vi "test BNR and BCD Parameters that Span Words.vi"(8 "error in":errorcluster, 11 "Loopback in":refnum<class "Loopback.lvclass">) -> (0 "error out":errorcluster, 3 "Loopback out":refnum<class "Loopback.lvclass">)   [LabVIEW 2020, in "Loopback.lvclass"]
uses:
  Loopback.lvclass
  C:/Users/nitest/Desktop/Git 2020/niveristand-custom-device-testing-tools/VeriStandTestCase/VeriStandTestCase.lvclass
  niveristand-custom-device-testing-tools/VeriStandTestUtilities/VeriStandTestUtilities.lvlib
  <vilib>/addons/_JKI Toolkits/VI Tester/TestCase.llb/TestCase.lvclass
  C:/Program Files (x86)/National Instruments/LabVIEW 2020/vi.lib/addons/_JKI Toolkits/VI Tester/TestCase.llb/TestCase.lvclass
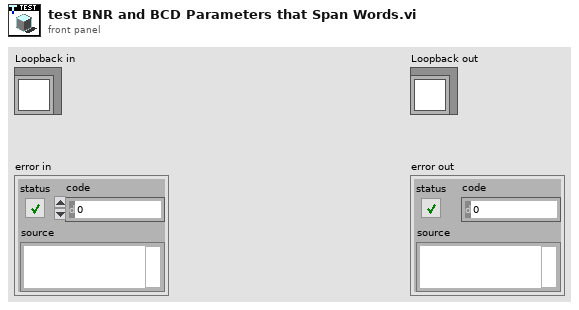
[diagram p1: front panel]
types:
  T1 = typedef "NI_VS Workspace ExecutionAPI.lvlib/WorkspaceAPI.ctl" = refnum<k24>
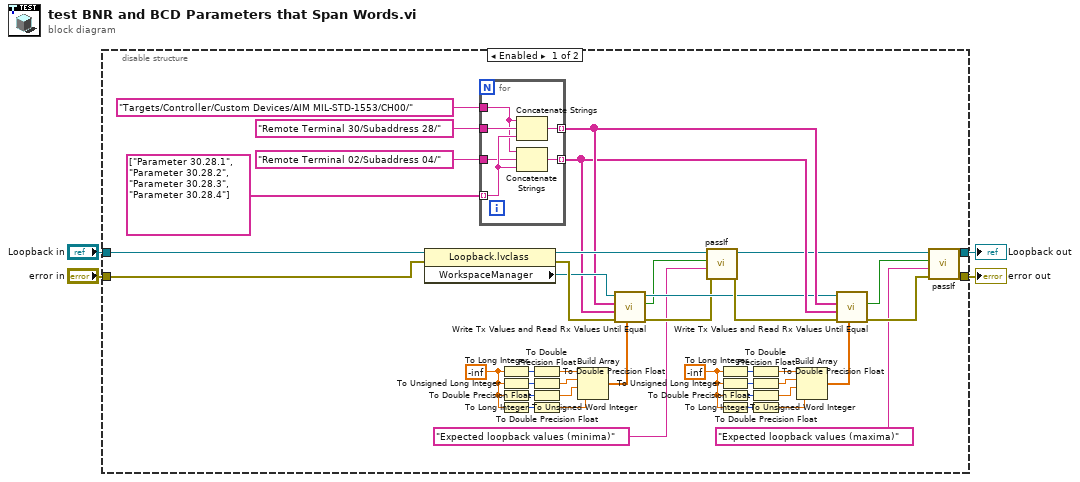
[diagram p0: block diagram]
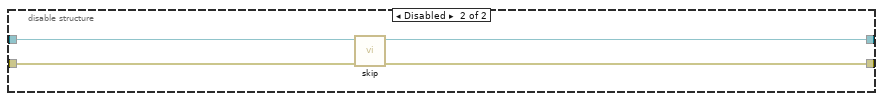
[diagram p2: hidden frame]
diagram:
  n1 = disable-structure shown="Enabled" {
    disable-tunnel: "Loopback in" -> [w46 w55]
    disable-tunnel: "error in" -> [w45 w56]
    disable-tunnel: [w32 w54] -> w2
    disable-tunnel: [w31 w53] -> w1
    frame Enabled {
      w13 = -inf
      w16 = -inf
      n2 = property class="Loopback.lvclass"(reference=w46, error in=w45) -> (reference out=w43:refnum<class "Loopback.lvclass">, error out=w44:errorcluster, "WorkspaceManager"=w42:T1)
      n3 = for {
        tunnel: "Remote Terminal 30/Subaddress 28/" ("Channel") -> [w51]
        tunnel: string[] ["Parameter 30.28.1", "Parameter 30.28.2", "Parameter 30.28.3", "Parameter 30.28.4"] ("Channels") -> [w50] mode=indexing
        tunnel: [w52] -> w39 mode=indexing
        tunnel: "Remote Terminal 02/Subaddress 04/" ("Channel") -> [w49]
        tunnel: [w48] -> w38 mode=indexing
        tunnel: "Targets/Controller/Custom Devices/AIM MIL-STD-1553/CH00/" ("base name for channel aliases") -> [w47]
        n4 = Concatenate Strings(w47, w51, w50) -> (w52:string)
        n5 = Concatenate Strings(w47, w49, w50) -> (w48:string)
      }
      n6 = To Long Integer(number=w16) -> (32bit integer=w24:i32)
      n7 = To Unsigned Long Integer(number=w16) -> (unsigned 32bit integer=w23:u32)
      n8 = To Long Integer(number=w16) -> (32bit integer=w22:i32)
      n9 = To Unsigned Word Integer(number=w16) -> (unsigned 16bit integer=w17:u16)
      n10 = To Double Precision Float(number=w24) -> (double precision float=w21:dbl)
      n11 = To Double Precision Float(number=w23) -> (double precision float=w20:dbl)
      n12 = To Double Precision Float(number=w22) -> (double precision float=w19:dbl)
      n13 = To Double Precision Float(number=w17) -> (double precision float=w15:dbl)
      n14 = Build Array(w21, w20, w19, w15) -> (w18:dbl[])
      n15 = call "Write Tx Values and Read Rx Values Until Equal.vi"("Tx values"=w18, "error in"=w44, "Rx aliases"=w38, "Tx aliases"=w39, "workspace manager in"=w42) -> ("error out"=w33:errorcluster, "values equal"=w34:bool, "workspace manager out"=w36:T1)  [unwired: 4 in]
      n16 = call-dynamic "passIf.vi"("error in (no error)"=w33, "message (\"\")"="Expected loopback values (minima)" ("message (\"\")"), "pass"=w34, "TestCase in"=w43) -> ("error out"=w37:errorcluster, "TestCase out"=w30:refnum<class "Loopback.lvclass">)  [unwired: 6 in]
      n17 = To Long Integer(number=w13) -> (32bit integer=w6:i32)
      n18 = To Unsigned Long Integer(number=w13) -> (unsigned 32bit integer=w7:u32)
      n19 = To Long Integer(number=w13) -> (32bit integer=w8:i32)
      n20 = To Unsigned Word Integer(number=w13) -> (unsigned 16bit integer=w12:u16)
      n21 = To Double Precision Float(number=w6) -> (double precision float=w9:dbl)
      n22 = To Double Precision Float(number=w7) -> (double precision float=w10:dbl)
      n23 = To Double Precision Float(number=w8) -> (double precision float=w11:dbl)
      n24 = To Double Precision Float(number=w12) -> (double precision float=w14:dbl)
      n25 = Build Array(w9, w10, w11, w14) -> (w5:dbl[])
      n26 = call "Write Tx Values and Read Rx Values Until Equal.vi"("Tx values"=w5, "error in"=w37, "Rx aliases"=w38, "Tx aliases"=w39, "workspace manager in"=w36) -> ("error out"=w40:errorcluster, "values equal"=w41:bool)  [unwired: 4 in, 1 out]
      n27 = call-dynamic "passIf.vi"("error in (no error)"=w40, "message (\"\")"="Expected loopback values (maxima)" ("message (\"\")"), "pass"=w41, "TestCase in"=w30) -> ("error out"=w32:errorcluster, "TestCase out"=w31:refnum<class "Loopback.lvclass">)  [unwired: 6 in]
    }
    frame Disabled {
      n28 = call <vilib>:"skip.vi"("error in (no error)"=w56, "TestCase in"=w55) -> ("error out"=w54:errorcluster, "TestCase out"=w53:refnum<class "Loopback.lvclass">)  [unwired: 8 in]
    }
  }
  "error out" <- w2
  "Loopback out" <- w1
